vi "latest2_version.vi"() -> ()   [LabVIEW 2024]
doc: "Use this template to build a producer/consumer design pattern. Use this template when you need to execute a process, such as data analysis, when a data source, such as a triggered acquisition, produces data at an uneven rate and you need to execute the process when the data becomes available."
uses:
  <vilib>/DAQmx/read.llb/DAQmx Read (Analog 2D DBL NChan NSamp).vi
  <vilib>/DAQmx/miscellaneous.llb/DAQmx Fill In Error Info.vi
  <vilib>/Utility/TDMS File Viewer/NI_TDMS File Viewer.lvlib
panel:
  in  "operation (0:open) 2":T1(ring)
  out "error out":errorcluster
  in  "file path":path
  in  "file format version (2.0)":enum16{"1.0", "2.0"}(ring)
  out "2D DBL":dbl[][](graph) caption="data"
  in  "STOP":bool caption="stop"
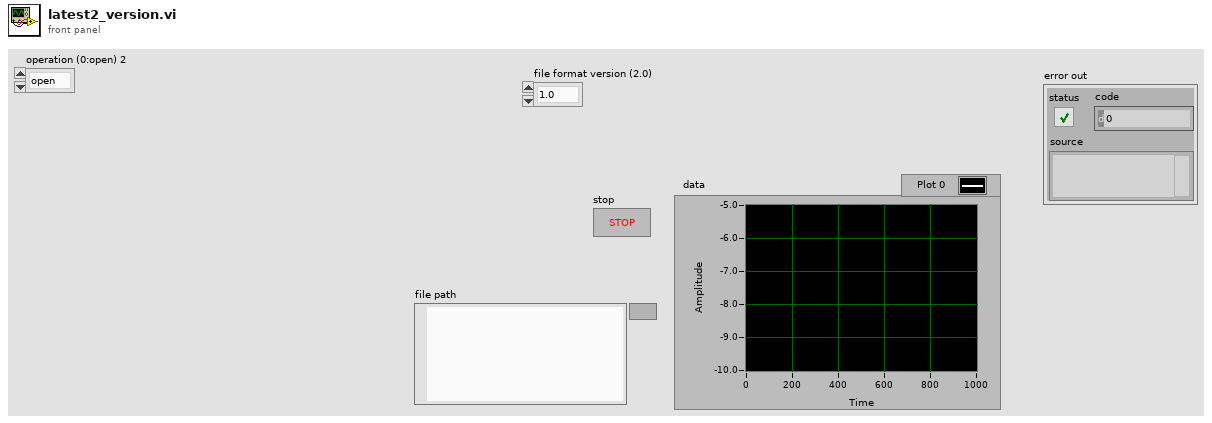
[diagram p1: front panel]
types:
  T1 = enum16{"open", "open or create", "create or replace", "create", "open (read-only)"}
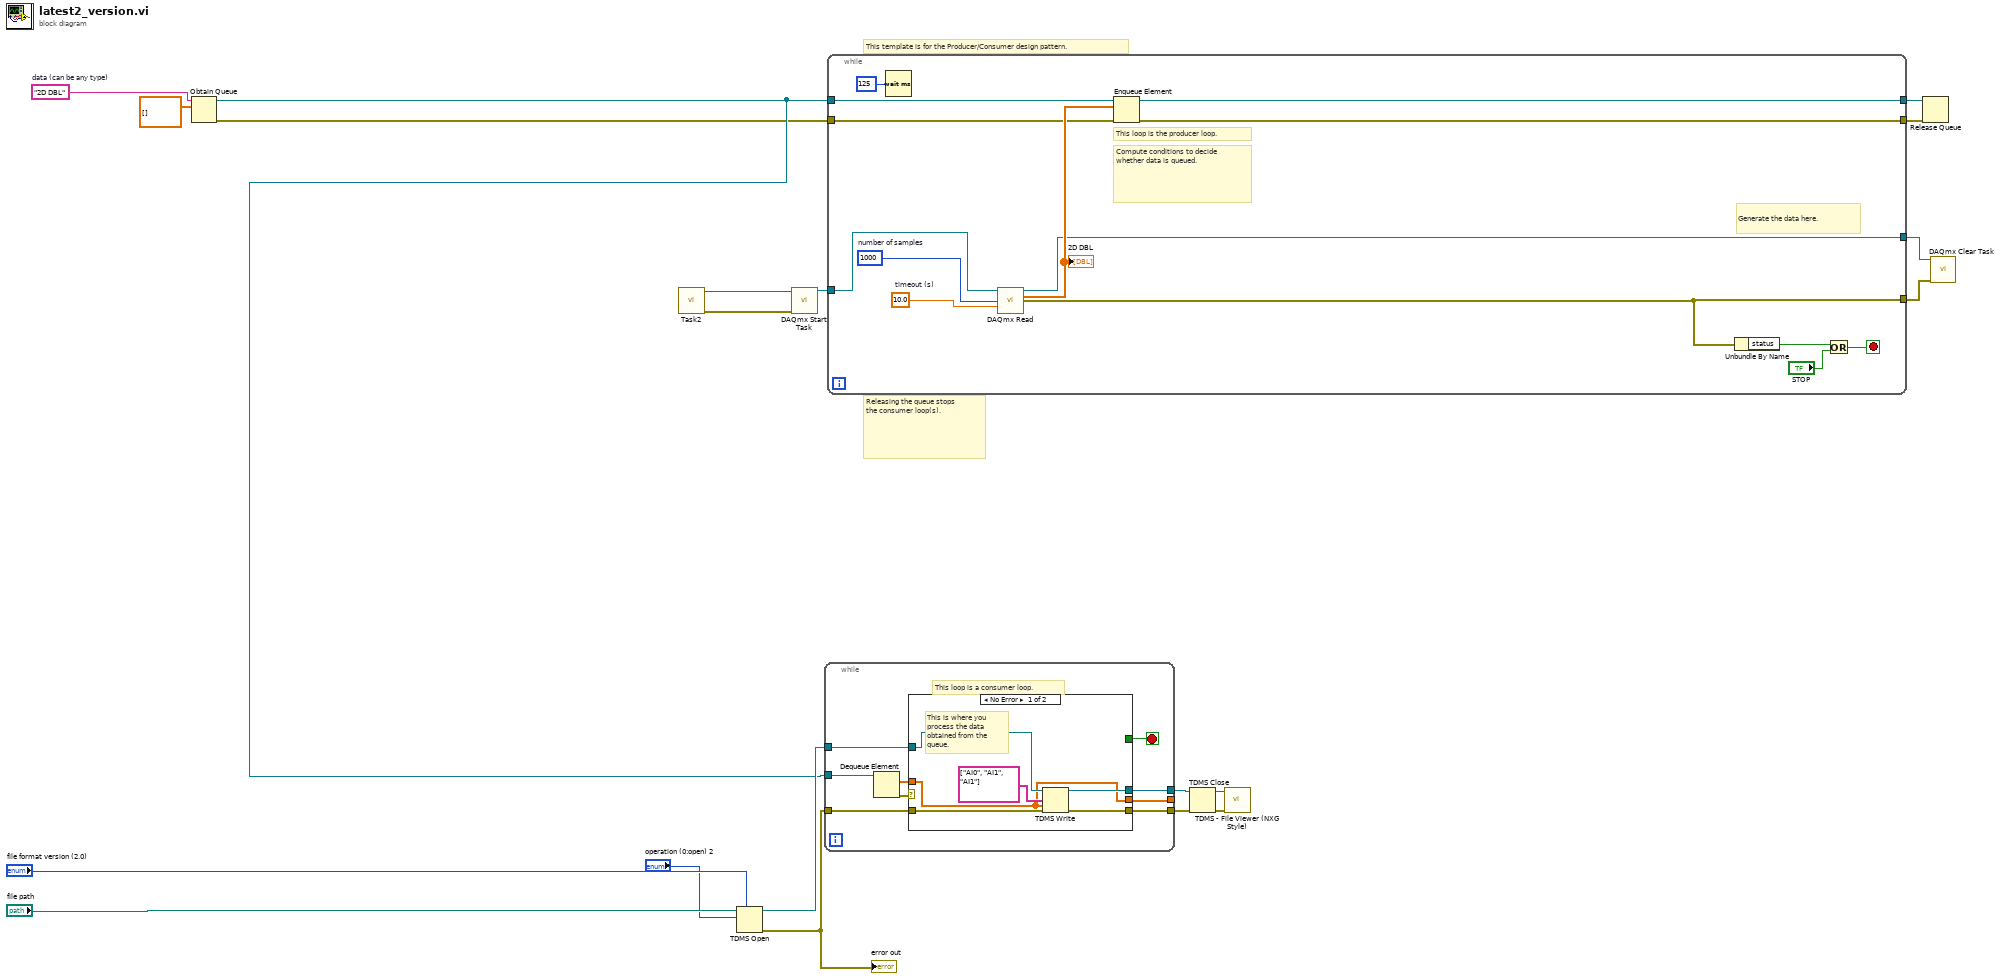
[diagram p0: block diagram]
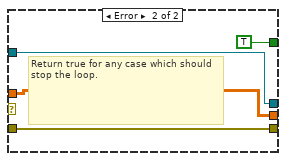
[diagram p2: hidden frame]
diagram:
  w19 = "2D DBL"  # data (can be any type)
  # "Releasing the queue stops the consumer loop(s)."
  # "This template is for the Producer/Consumer design pattern."
  n1 = Obtain Queue(name (unnamed)=w19, element data type=dbl[][] []) -> (queue out=w5:refnum<queue>, error out=w4:errorcluster)  [unwired: 3 in, 1 out]
  n2 = call "Task2.vi"() -> ("error out"=w2:errorcluster, "task out"=w3:refnum<k21>)  [unwired: 10 in]
  n3 = TDMS Open(7:"file format version (2.0)", 10:"operation (0:open) 2", 11:"file path") -> (0:w14:errorcluster, 3:w13:refnum<k34>)  [unwired: 4 in]
  "error out" <- w14
  n4 = call <vilib>:"DAQmx Start Task.vi"("task/channels in"=w3, "error in"=w2) -> ("task out"=w20:refnum<k21>)  [unwired: 12 in, 1 out]
  n5 = while {
    tunnel: w5 -> [w29]
    tunnel: w14 -> [w25]
    tunnel: w13 -> [w24]
    tunnel: [w23] -> w11
    tunnel: [w22] -> w12
    tunnel: [w21] -> _
    stop <- w26 stop-if-true
    # "This loop is a consumer loop."
    n6 = Dequeue Element(queue=w29) -> (element=w27:dbl[][], error out=w28:errorcluster)  [unwired: 2 in, 2 out]
    n7 = case shown="No Error" w28 {
      tunnel: w27 -> [w30 w36]
      tunnel: [_ TRUE] -> w26
      tunnel: w25 -> [w35 w38]
      tunnel: w24 -> [w34 w37]
      tunnel: [w33 w37] -> w23
      tunnel: [w32 w38] -> w22
      tunnel: [w30 w36] -> w21
      frame No Error {
        # "This is where you process the data obtained from the queue."
        n8 = TDMS Write(0:w34, 7:string[] ["AI0", "AI1", "AI1"] ("channel name(s) in (Untitled)"), 9:w30, 11:w35) -> (4:w33:refnum<k34>, 15:w32:errorcluster)  [unwired: 2 in, 2 out]
      }
      frame Error {
        # "Return true for any case which should stop the loop."
      }
    }
  }
  n9 = while {
    tunnel: w20 -> [w52]
    tunnel: [w48] -> w16
    tunnel: [w47] -> w15
    tunnel: [w43] -> w7
    tunnel: [w42] -> w6
    tunnel: w5 -> [w41]
    tunnel: w4 -> [w40]
    stop <- w49 stop-if-true
    w44 = 10.0  # timeout (s)
    w51 = 1000  # number of samples
    # "Generate the data here."
    # "Compute conditions to decide whether data is queued."
    # "This loop is the producer loop."
    n10 = Wait (ms)(milliseconds to wait=u32 125) -> ()  [unwired: 1 out]
    n11 = call-poly <vilib>:"DAQmx Read.vi"("task/channels in"=w52, "number of samples per channel"=w51, "timeout"=w44) -> ("task out"=w43:refnum<k21>, "data"=w50:dbl[][], "error out"=w42:errorcluster)  [unwired: 10 in]
    "2D DBL" <- w50
    n12 = Enqueue Element(queue=w41, element=w50, error in (no error)=w40) -> (queue out=w48:refnum<queue>, error out=w47:errorcluster)  [unwired: 1 in, 1 out]
    n13 = Unbundle By Name(w42) -> ("status"=w45:bool)
    n14 = Or(x=w45, y="STOP") -> (x .or. y?=w49:bool)
  }
  n15 = TDMS Close(8:w12, 11:w11) -> (0:w9:errorcluster, 3:w8:path)
  n16 = call <vilib>:"TDMS - File Viewer (NXG Style).vi"("error in"=w9, "file in"=w8) -> ()  [unwired: 8 in, 2 out]
  n17 = Release Queue(queue=w16, error in (no error)=w15) -> ()  [unwired: 1 in, 3 out]
  n18 = call <vilib>:"DAQmx Clear Task.vi"("task in"=w7, "error in"=w6) -> ()  [unwired: 13 in, 1 out]
